vi "Data_Read_Write.vi"(1 "name":string, 2 "Data":string, 3 "error initialize":errorcluster) -> (9 "error out":errorcluster)   [LabVIEW 2015]
uses:
  Data Read Write Control.ctl
panel:
  in  "Data Read Write Control":T1
  out "cancelled 2":bool
  out "path":path
  out "cancelled":bool
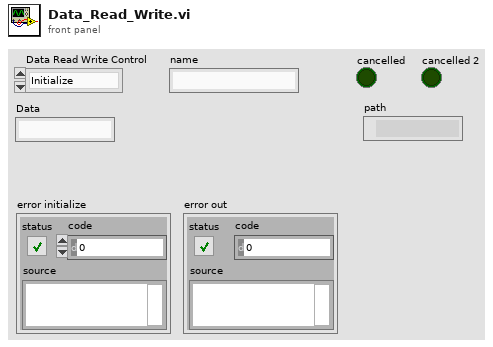
[diagram p1: front panel]
types:
  T1 = typedef "Data Read Write Control.ctl" = enum16{"Initialize", "Read", "Write", "Close"}
  T2 = enum16{"open", "replace", "create", "open or create", "replace or create", "replace or create with confirmation"}
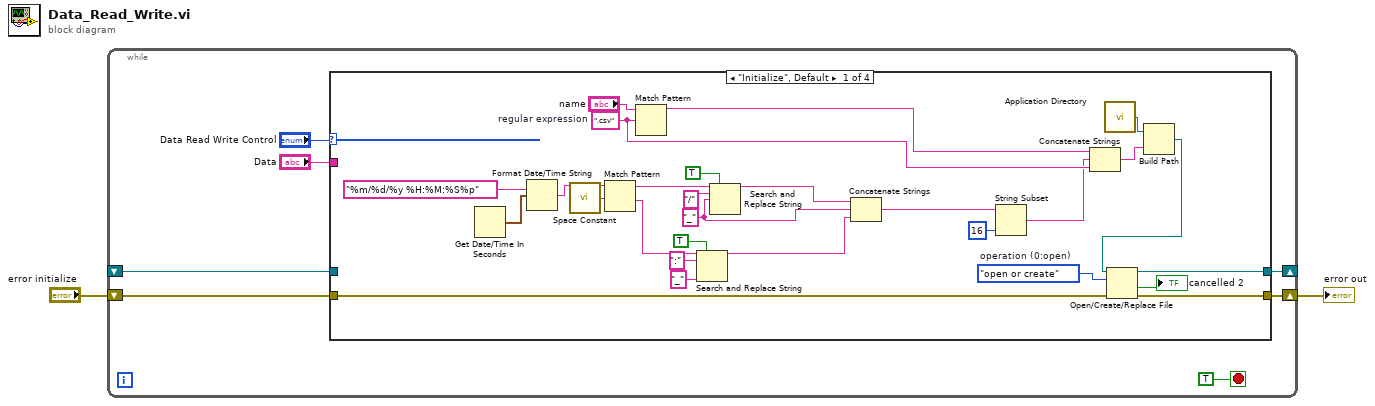
[diagram p0: block diagram]
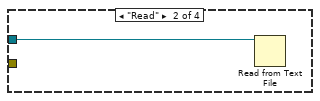
[diagram p2: hidden frame]
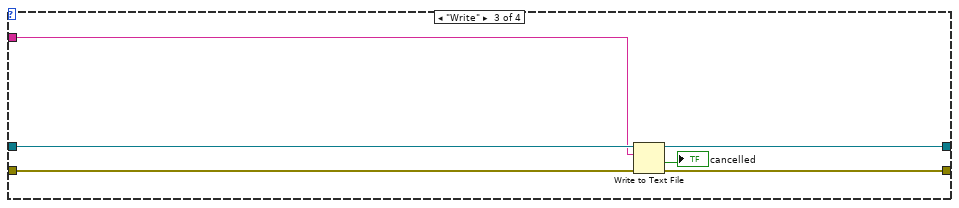
[diagram p3: hidden frame]
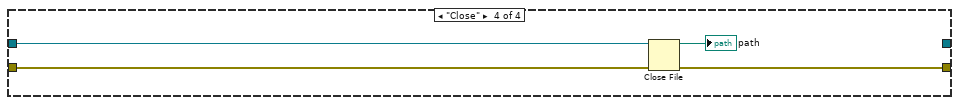
[diagram p4: hidden frame]
diagram:
  n1 = while {
    shift-right: [w7] -> w2
    shift-left: "error initialize" -> [w6]
    shift-right: [w5] -> _
    shift-left: _ -> [w4]
    stop <- TRUE stop-if-true
    n2 = case shown="\"Initialize\", Default" "Data Read Write Control" {
      tunnel: "Data" -> [_ _ w40 _]
      tunnel: [w37 _ w44 w48] -> w7
      tunnel: w6 -> [w36 _ w43 w47]
      tunnel: [w35 _ w42 _] -> w5
      tunnel: w4 -> [_ w38 w41 w46]
      frame "Initialize", Default {
        w10 = "_" ("replace string (\"\")")
        w13 = ".csv"  # regular expression
        w32 = T2."open or create"  # operation (0:open)
        n3 = Get Date/Time In Seconds() -> (seconds since 1Jan1904=w30:timestamp)
        n4 = Format Date/Time String(time format string (%c)="%m/%d/%y %H:%M:%S%p", seconds (now)=w30) -> (date/time string=w26:string)  [unwired: 1 in]
        n5 = call <vilib>:"Space Constant.vi"() -> ("String"=w25:string)
        n6 = Match Pattern(string=w26, regular expression=w25) -> (before substring=w24:string, after substring=w22:string)  [unwired: 1 in, 2 out]
        n7 = Match Pattern(string="name", regular expression=w13) -> (before substring=w11:string)  [unwired: 1 in, 3 out]
        n8 = Search and Replace String(replace all?=TRUE ("replace all? (F)"), input string=w22, search string=":", replace string="_" ("replace string (\"\")")) -> (result string=w18:string)  [unwired: 4 in, 3 out]
        n9 = Search and Replace String(replace all?=TRUE ("replace all? (F)"), input string=w24, search string="/", replace string=w10) -> (result string=w19:string)  [unwired: 4 in, 3 out]
        n10 = Concatenate Strings "Concatenate Strings"(w19, w10, w18) -> (w15:string)
        n11 = String Subset(string=w15, length (rest)=16 ("length (rest)")) -> (substring=w12:string)  [unwired: 1 in]
        n12 = Concatenate Strings "Concatenate Strings"(w11, w12, w13) -> (w27:string)
        n13 = call <vilib>:"Application Directory.vi"() -> ("Application Directory"=w31:path)
        n14 = Build Path(base path=w31, name or relative path=w27) -> (appended path=w34:path)
        n15 = Open/Create/Replace File(file path (use dialog)=w34, error in=w36, operation (0:open)=w32) -> (refnum out=w35:refnum<file>, cancelled=→"cancelled 2":bool, error out=w37:errorcluster)  [unwired: 3 in]
      }
      frame "Read" {
        n16 = Read from Text File(file (use dialog)=w38) -> ()  [unwired: 3 in, 4 out]
      }
      frame "Write" {
        n17 = Write to Text File(file (use dialog)=w41, text=w40, error in=w43) -> (refnum out=w42:refnum<file>, cancelled=→"cancelled":bool, error out=w44:errorcluster)  [unwired: 1 in]
      }
      frame "Close" {
        n18 = Close File(refnum=w46, error in=w47) -> (path=→"path":path, error out=w48:errorcluster)
      }
    }
  }
  "error out" <- w2
